vi "Find All Readers of Data.vi"(8 "error in (no error)":errorcluster, 10 "Full Element Name":string[](array[string]), 11 "JKI SM in":refnum<class "JKI SM.lvclass">) -> (0 "error out":errorcluster, 2 "NamedUnbundlers":refnum<vi>[](array[refnum]), 3 "JKI SM out":refnum<class "JKI SM.lvclass">)   [LabVIEW 2020, in "JKI State Machine API.lvlib" / "JKI SM.lvclass"]
uses:
  JKI SM.lvclass
  <vilib>/Utility/traverseref.llb/TRef TravTarget.ctl
  JKI SM.lvclass/JKI SM.ctl
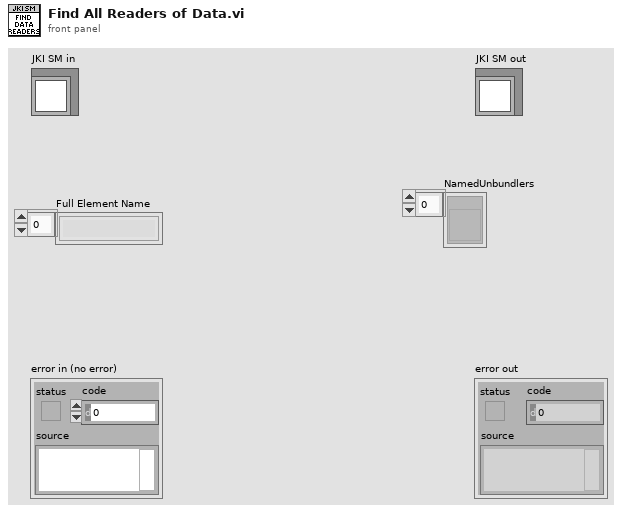
[diagram p1: front panel]
types:
  T1 = typedef "TRef TravTarget.ctl" = enum16{"FP", "BD", "Other"}
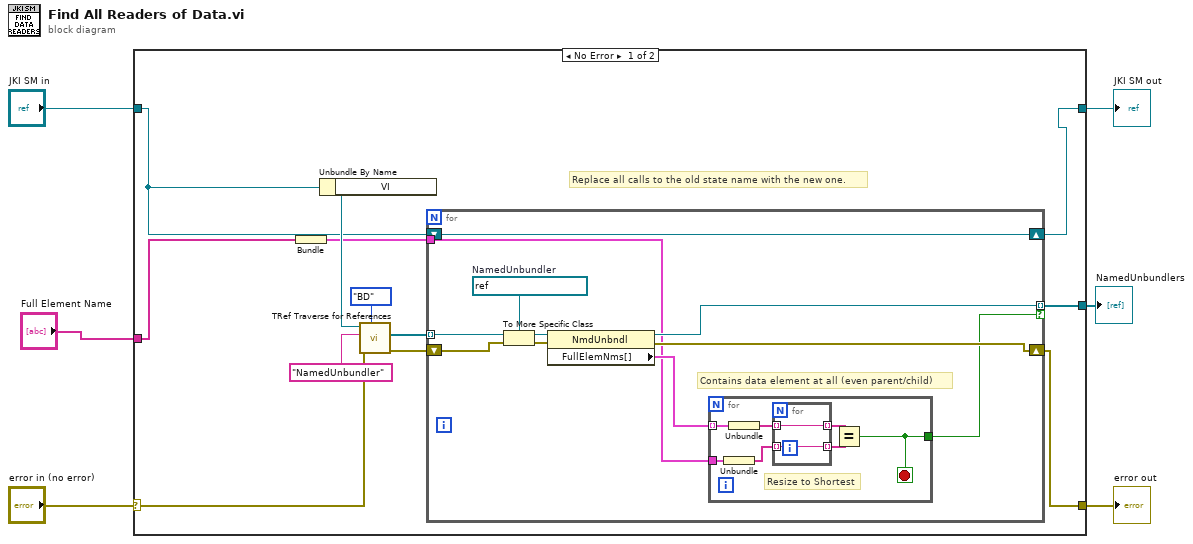
[diagram p0: block diagram]
diagram:
  n1 = case shown="No Error" "error in (no error)" {
    selector: "error in (no error)" -> [w11 w40]
    tunnel: [w10 w40] -> w5
    tunnel: [w12 w39] -> w3
    tunnel: "JKI SM in" -> [w13 w39]
    tunnel: "Full Element Name" -> [w7 _]
    tunnel: [w9 _] -> w1
    frame No Error {
      # "Replace all calls to the old state name with the new one."
      n2 = Bundle("Full Element Name"=w7) -> (w8:cluster{"Full Element Name":string[]})  [unwired: 1 in]
      n3 = Unbundle By Name(w13) -> ("VI"=w14:refnum<vi>)
      n4 = call <vilib>:"TRef Traverse for References.vi"("Traverse Target"=TRef_TravTarget."BD", "error in (no error)"=w11, "Class Name"="NamedUnbundler", "VI Refnum"=w14) -> ("error out"=w15:errorcluster, "References"=w16:refnum<vi>[])  [unwired: 1 in, 5 out]
      n5 = for {
        tunnel: w16 -> [w29] mode=indexing
        tunnel: w8 -> [w19]
        shift-right: [w25] -> w12
        shift-left: w13 -> [w25]
        shift-right: [w22] -> w10
        shift-left: w15 -> [w27]
        tunnel: [w23] -> w9 mode=indexing if=w20
        w24 = refnum<vi> refnum  # NamedUnbundler
        # "Contains data element at all (even parent/child)"
        n6 = To More Specific Class(target class=w24, reference=w29, error in=w27) -> (specific class reference=w28:refnum<vi>, error out=w26:errorcluster)
        n7 = property class="NmdUnbndl"(reference=w28, error in=w26) -> (reference out=w23:refnum<vi>, error out=w22:errorcluster, "FullElemNms[]"=w21:cluster{string[]}[])
        n8 = for {
          tunnel: w21 -> [w36] mode=indexing
          tunnel: [w32] -> w20
          tunnel: w19 -> [w31]
          stop <- w32 stop-if-true
          # "Resize to Shortest"
          n9 = Unbundle(w31) -> ("Full Element Name"=w30:string[])
          n10 = Unbundle(w36) -> (w35:string[])
          n11 = for {
            tunnel: w35 -> [w37] mode=indexing
            tunnel: w30 -> [w38] mode=indexing
            tunnel: [w38] -> w33 mode=indexing
            tunnel: [w37] -> w34 mode=indexing
          }
          n12 = Equal?(x=w34, y=w33) -> (x = y?=w32:bool)
        }
      }
    }
    frame Error {
    }
  }
  "error out" <- w5
  "JKI SM out" <- w3
  "NamedUnbundlers" <- w1
